vi "niRFUtil CONV Complex Waveform to Complex WDT.vi"(7 "Complex Waveform":T2 {"y" format="%.2f"; "dx" format="%^.2e"; "x0" format="%^.2e"}) -> (8 "Complex WDT":T1)   [LabVIEW 2015, in "niRFUtil.lvlib"]
uses:
  niRFUtil.lvlib
  Includes/niRFUtil INC Complex Waveform.ctl
  Includes/niRFUtil INC Complex Array.ctl
  Includes/niRFUtil INC Complex WDT.ctl
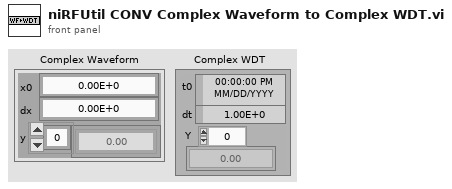
[diagram p1: front panel]
types:
  T1 = typedef "niRFUtil.lvlib/niRFUtil INC Complex WDT.ctl" = waveform(csg)
  T2 = typedef "niRFUtil.lvlib/niRFUtil INC Complex Waveform.ctl" = cluster{"x0":dbl, "dx":dbl, "y":T3}
  T3 = typedef "niRFUtil.lvlib/niRFUtil INC Complex Array.ctl" = csg[]
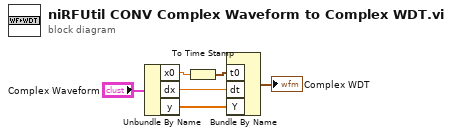
[diagram p0: block diagram]
diagram:
  n1 = Unbundle By Name("Complex Waveform") -> ("x0"=w4:dbl, "dx"=w2:dbl, "y"=w1:T3)
  n2 = To Time Stamp(1:w4) -> (0:w3:timestamp)
  n3 = Bundle By Name("t0"=w3, "dt"=w2, "Y"=w1) -> (→"Complex WDT":waveform(csg))  [unwired: 1 out]
